vi "dequeue state & data.vi"(8 "error in (no error)":errorcluster, 9 "timeout in ms (-1)":i32=-1, 11 "queue in":refnum<queue>) -> (0 "error out":errorcluster, 1 "State Data":variant, 2 "State":string, 3 "queue out":refnum<queue>)   [LabVIEW 2015, in "Ev Queued SM API.lvlib"]
doc: "This VI extracts the message from the queue. In case an error is entered by the <b>error in</b> input,\nthe case selector in <b>Main.vi</b> will receive the <b>Shutdown</b> status, which causes the machine to shut down.\nIf you ever change the name <b>Shutdown</b> to something else, you must do the same in the case structure of <b>Main.vi</b>."
uses:
  Ev Queued SM API.lvlib
  controls/State & Data Cluster.ctl
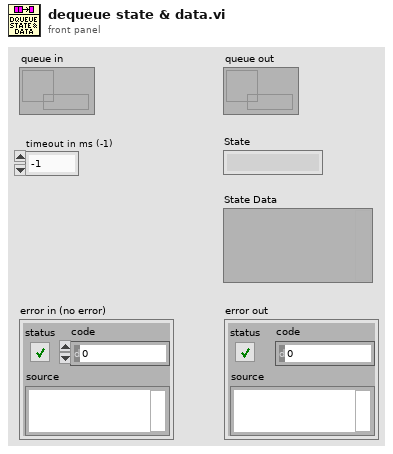
[diagram p1: front panel]
types:
  T1 = typedef "Ev Queued SM API.lvlib/State & Data Cluster.ctl" = cluster{"State":string, "Data":variant}
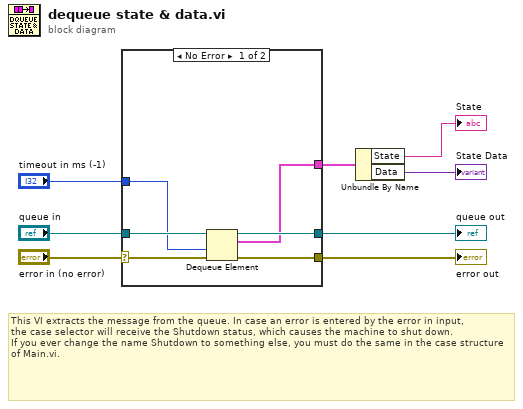
[diagram p0: block diagram]
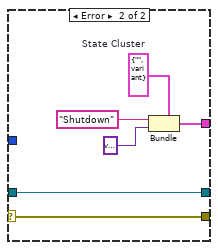
[diagram p2: hidden frame]
diagram:
  # "This VI extracts the message from the queue. In case an error is entered by the error in input,\nthe case selector will receive the Shutdown status, which causes the machine to shut down.\nIf you ever change the name Shutdown to something else, you must do the same in the case structure of Main.vi."
  n1 = case shown="No Error" "error in (no error)" {
    selector: "error in (no error)" -> [w10 w20]
    tunnel: [w14 w20] -> w8
    tunnel: "queue in" -> [w13 w19]
    tunnel: [w12 w19] -> w5
    tunnel: [w11 w16] -> w4
    tunnel: "timeout in ms (-1)" -> [w9 _]
    frame No Error {
      n2 = Dequeue Element(queue=w13, timeout in ms (-1)=w9, error in (no error)=w10) -> (queue out=w12:refnum<queue>, element=w11:T1, error out=w14:errorcluster)  [unwired: 1 out]
    }
    frame Error {
      w15 = T1 {"State"="", "Data"=variant}  # State Cluster
      n3 = Bundle(cluster=w15, "State"="Shutdown", "Data"=variant) -> (w16:T1)
    }
  }
  "error out" <- w8
  "queue out" <- w5
  n4 = Unbundle By Name(w4) -> ("State"=→"State":string, "Data"=→"State Data":variant)
